vi "atcs_getEvent_TelescopeInPosition.vi"(8 "error in (no error)":errorcluster, 11 "logevent_TelescopeInPosition_Ctl":T1) -> (0 "error out":errorcluster, 2 "function return":i32, 3 "logevent_TelescopeInPosition_Ctl out":T1)   [LabVIEW 2016, in "SALLV_atcs.lvlib"]
doc: "int atcs_shm_getEvent_TelescopeInPositionLV(atcs_logevent_TelescopeInPositionLV *logevent_TelescopeInPosition_Ctl );"
uses:
  SALLV_atcs.lvlib
  DataTypes/logevent_TelescopeInPosition.ctl
  SALLV_atcs.so
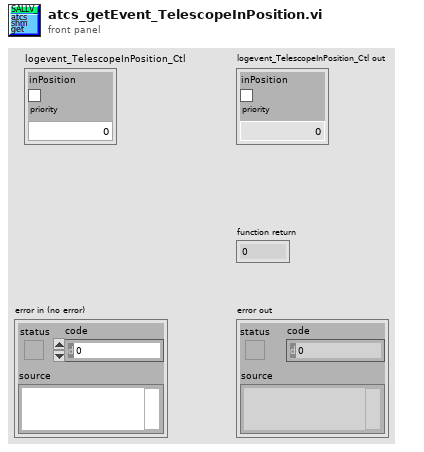
[diagram p1: front panel]
types:
  T1 = typedef "SALLV_atcs.lvlib/logevent_TelescopeInPosition.ctl" = cluster{"inPosition":bool, "priority":i32}
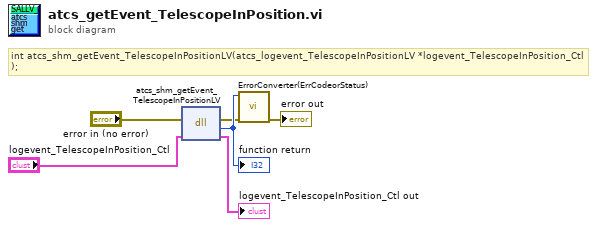
[diagram p0: block diagram]
diagram:
  # "int atcs_shm_getEvent_TelescopeInPositionLV(atcs_logevent_TelescopeInPositionLV *logevent_TelescopeInPosition_Ctl );"
  n1 = dll-call lib="home/andres/Desktop/SALLV_atcs/SALLV_atcs.*" fn="atcs_shm_getEvent_TelescopeInPositionLV"(error in="error in (no error)", "logevent_TelescopeInPosition_Ctl"="logevent_TelescopeInPosition_Ctl") -> (error out=w2:errorcluster, w6:i32, "logevent_TelescopeInPosition_Ctl"=→"logevent_TelescopeInPosition_Ctl out":T1)  [unwired: 2 in, 1 out]
  "function return" <- w6
  n2 = call "ErrorConverter(ErrCodeorStatus).vi"("error in (no error)"=w2, "error code"=w6) -> ("error out"=→"error out":errorcluster)  [unwired: 9 in]
